vi "xio.delete_lua.vi"(5 "LuaVIEW reference":T1) -> (15 "error out":errorcluster)   [LabVIEW 2012]
doc: "Delete a file or an empty directory. To recursively delete a directory tree, use the following function definition:\n<pre><code>function xio.deletetree(path)\n local files,dirs=xio.listdir(path)\n for i,d in ipairs(dirs) do\n xio.deletetree(d)\n end\n for i,f in ipairs(files) do\n xio.delete(f)\n end\n xio.delete(path)\nend</code></pre>\nParameters:\nstr:path\nErrors:\nFile or directory not found.\nFile in use.\nDirectory not empty.\nAccess denied."
uses:
  typedefs/t_LuaVIEW Reference.ctl
  subvis/private/LuaVIEW Pull (path).vi
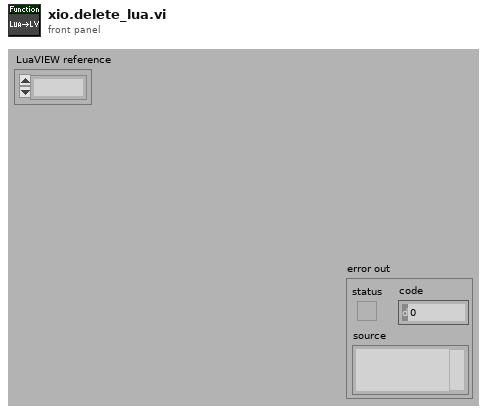
[diagram p1: front panel]
types:
  T1 = typedef "t_LuaVIEW Reference.ctl" = refnum<k1>
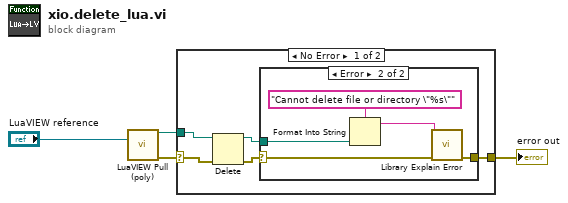
[diagram p0: block diagram]
diagram:
  n1 = call-poly "LuaVIEW Pull (poly).vi"("LuaVIEW reference in"="LuaVIEW reference") -> ("path"=w4:path, "error out"=w3:errorcluster)  [unwired: 12 in, 1 out]
  n2 = case shown="No Error" w3 {
    selector: w3 -> [w9 w16]
    tunnel: w4 -> [w6 _]
    tunnel: [w7 w16] -> w2
    frame No Error {
      n3 = Delete(path (use dialog)=w6, error in=w9) -> (deleted path=w5:path, error out=w8:errorcluster)  [unwired: 3 in, 1 out]
      n4 = case shown="Error" w8 {
        selector: w8 -> [w10 w15]
        tunnel: [w10 w14] -> w7
        tunnel: w5 -> [_ w11]
        frame No Error {
        }
        frame Error {
          n5 = Format Into String(format string="Cannot delete file or directory \"%s\"", w11) -> (resulting string=w13:string)  [unwired: 2 in, 1 out]
          n6 = call "Library Explain Error.vi"("explanation prefix (none)"=w13, "error in (no error)"=w15) -> ("explained error"=w14:errorcluster)  [unwired: 13 in]
        }
      }
    }
    frame Error {
    }
  }
  "error out" <- w2
